vi "Practica 04.vi"() -> ()   [LabVIEW 2011]
panel:
  in  "OK Button 2":bool
  in  "D":dbl
  in  "I":dbl
  in  "P":dbl
  in  "Control de Velocidad (RPM)":i32(knob) scale=-3000.0..3000.0
  out "RPM's":dbl(knob) scale=0.0..3000.0
  out "Alarma !":bool
  in  "OK Button":bool
  in  "SERVO ON":bool
  # "Deslizador Lineal UTN"
  # "CONTOL DE VELOCIDAD"
  # "CONTROL DE VELOCIDAD - Lazo Cerrado"
  # "Variables de Control"
  # "1. Encender el servomotor"
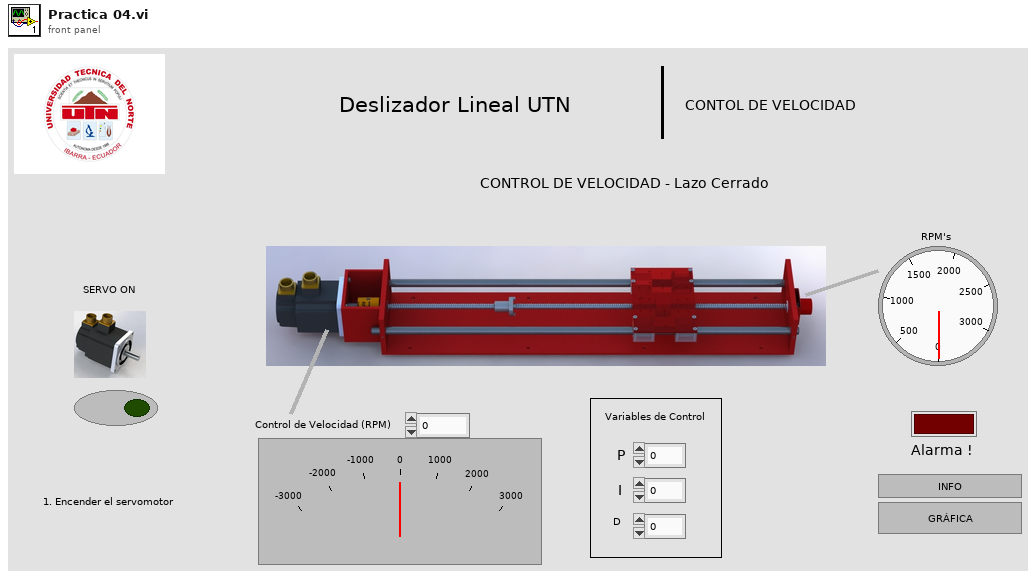
[diagram p1: front panel]
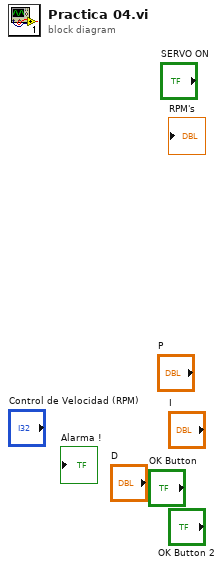
[diagram p0: block diagram]
diagram:
